vi "Contour Analysis.vi"() -> ()   [LabVIEW 2014]
doc: "This example shows a contour analysis of a painted object. The contour of the paint boundary is extracted, and the curvature of this contour is displayed. Adjusting the kernel width will change the curvature profile to highlight curves at different scales."
uses:
  <vilib>/vision/Contour.llb/IMAQ Connect Range Setting.ctl
  <vilib>/vision/Contour.llb/IMAQ Contour Curve Extraction.ctl
  <vilib>/vision/NI_Vision_Development_Module.lvlib
panel:
  out "Curvature Profile":dbl[](graph)
  in  "Stop":bool
  out "Image":T1(plugin-control)
  in  "Delay (s.)":dbl(slide)=1.4899328859060401 scale=0.0..3.0
  # "Overview: Demonstrates how to use the IMAQ Extract Contour function to extract the contour of edges and then use IMAQ Compute Curvature to calculate the curvature of the extracted contour and plot the curvature profile.\nRequirements: Vision Development Software.\nInstructions:  Run the VI."
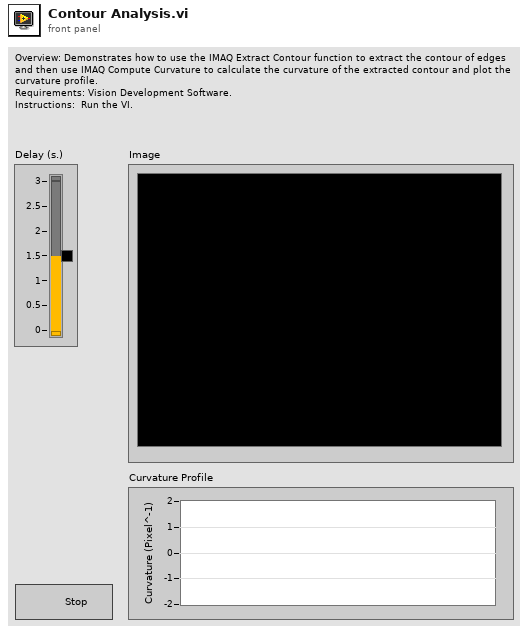
[diagram p1: front panel]
types:
  T1 = typedef "IMAQ Image.ctl" = refnum<image>
  T2 = typedef "IMAQ Rectangle" = cluster{"Left":i32, "Top":i32, "Right":i32, "Bottom":i32, "Rotation":dbl}
  T3 = typedef "ROI Descriptor" = cluster{"Global Rectangle":i32[], "Contours":cluster{"ID":enum32{"External", "Internal"}, "Type":u32, "Coordinates":i32[]}[]}
  T4 = typedef "IMAQ Connect Range Setting.ctl" = cluster{"Match Constraints":u32, "Min":dbl, "Max":dbl}
  T5 = cluster{"Overlay?":bool, "Color":u32, "Width":u32, "Maintain Width?":bool}
  T6 = enum16{"Closest To Search Start", "Maximum Length", "Strongest Mean Gradient Change"}
  T7 = enum16{"Rect Left To Right", "Rect Right To Left", "Rect Top To Bottom", "Rect Bottom To Top", "Annulus Inner To Outer", "Annulus Outer To Inner", "Annulus Start Angle To End Angle", "Annulus End Angle To Start Angle"}
  T8 = typedef "IMAQ Contour Curve Extraction.ctl" = cluster{"Extraction Mode":u32, "Edge Threshold":i32, "Edge Filter Size":u32, "Min Length":i32, "Search Step Size":i32, "Max Endpoint Gap":i32, "Subpixel":bool}
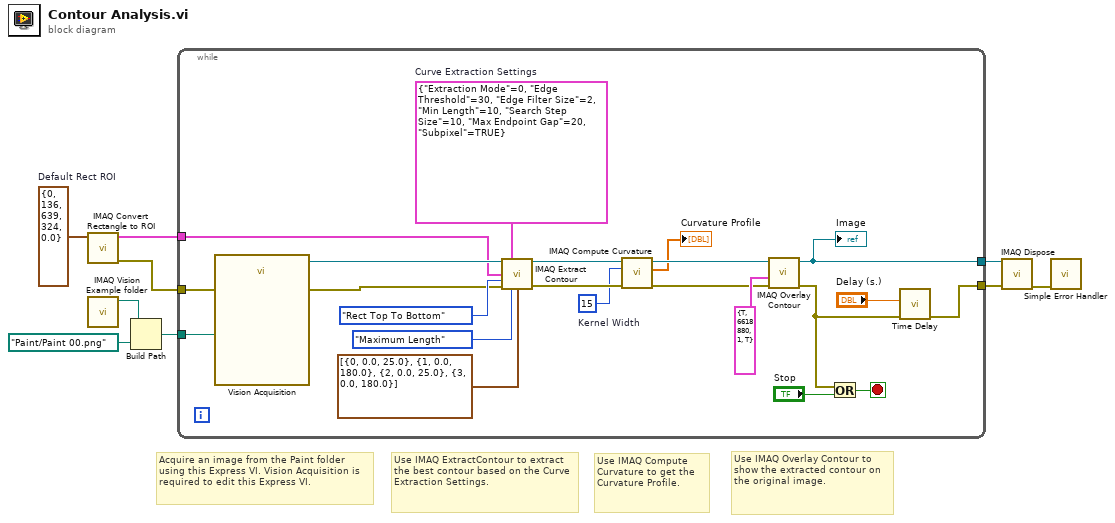
[diagram p0: block diagram]
diagram:
  w4 = T2 {"Left"=0, "Top"=136, "Right"=639, "Bottom"=324, "Rotation"=0.0}  # Default Rect ROI
  # "Acquire an image from the Paint folder using this Express VI. Vision Acquisition is required to edit this Express VI."
  # "Use IMAQ Overlay Contour to show the extracted contour on the original image."
  # "Use IMAQ Compute Curvature to get the Curvature Profile."
  # "Use IMAQ ExtractContour to extract the best contour based on the Curve Extraction Settings."
  n1 = call "IMAQ Convert Rectangle to ROI"("Rectangle"=w4) -> ("error out"=w2:errorcluster, "ROI Descriptor"=w3:T3)  [unwired: 8 in]
  n2 = call "IMAQ Vision Example folder.vi"() -> ("Example Image Path"=w6:path)  [unwired: 11 in]
  n3 = Build Path(base path=w6, name or relative path=path "Paint/Paint 00.png") -> (appended path=w5:path)
  n4 = while {
    tunnel: [w20] -> w9
    tunnel: [w10] -> w8
    tunnel: w5 -> [w15]
    tunnel: w3 -> [w14]
    tunnel: w2 -> [w13]
    stop <- w16 stop-if-true
    w24 = u32 15  # Kernel Width
    w23 = T8 {"Extraction Mode"=0, "Edge Threshold"=30, "Edge Filter Size"=2, "Min Length"=10, "Search Step Size"=10, "Max Endpoint Gap"=20, "Subpixel"=TRUE}  # Curve Extraction Settings
    n5 = call "Vision Acquisition"("Image Path"=w15, "error in"=w13) -> ("Image Out"=w22:T1, "error out"=w21:errorcluster)  [unwired: 23 in, 1 out]
    n6 = call "IMAQ Extract Contour"("Source Image"=w22, "Curve Extraction"=w23, "ROI Descriptor"=w14, "Search Direction"=T7."Rect Top To Bottom", "error in (no error)"=w21, "Contour Selection"=T6."Maximum Length", "Curve Connection"=T4[] [{"Match Constraints"=0, "Min"=0.0, "Max"=25.0}, {"Match Constraints"=1, "Min"=0.0, "Max"=180.0}, {"Match Constraints"=2, "Min"=0.0, "Max"=25.0}, {"Match Constraints"=3, "Min"=0.0, "Max"=180.0}]) -> ("Source Image Out"=w12:T1, "error out"=w27:errorcluster)  [unwired: 1 in, 6 out]
    n7 = call "IMAQ Compute Curvature"("error in (no error)"=w27, "Kernel Width"=w24, "Contour Image"=w12) -> ("error out"=w26:errorcluster, "Curvature Profile (pixel)"=→"Curvature Profile":dbl[], "Contour Image Out (dup)"=w25:T1)  [unwired: 6 out]
    n8 = call "IMAQ Overlay Contour"("error in (no error)"=w26, "Contour Points Settings"=T5 {"Overlay?"=TRUE, "Color"=6618880, "Width"=1, "Maintain Width?"=TRUE}, "Image"=w25) -> ("error out"=w18:errorcluster, "Image Out"=w20:T1)  [unwired: 3 in, 4 out]
    "Image" <- w20
    n9 = Or(x=w18, y="Stop") -> (x .or. y?=w16:bool)
    n10 = call "Time Delay"("error in (no error)"=w18, "Delay Time (s)"="Delay (s.)") -> ("error out"=w10:errorcluster)  [unwired: 9 in]
  }
  n11 = call "IMAQ Dispose"("Image"=w9, "error in (no error)"=w8) -> ("error out"=w1:errorcluster)  [unwired: 1 in, 3 out]
  n12 = call <vilib>:"Simple Error Handler.vi"("error in (no error)"=w1) -> ()  [unwired: 4 in, 5 out]
